vi "Insert Menu Items.vi"(6 "after item":string, 7 "menu tag":string, 8 "error in (no error)":errorcluster, 9 "item tags":string[](array[string]), 10 "item names":string[](array[string]), 11 "Menu in":refnum<class "Menu.lvclass">) -> (0 "error out":errorcluster, 1 "item tags out":string[](array[string]), 3 "Menu out":refnum<class "Menu.lvclass">)   [LabVIEW 2021, in "Menu.lvlib" / "Menu.lvclass"]
uses:
  Menu.lvclass
  <vilib>/Utility/miscctls.llb/LVMapReplaceAction.ctl
  <vilib>/Utility/miscctls.llb/LVPoint32TypeDef.ctl
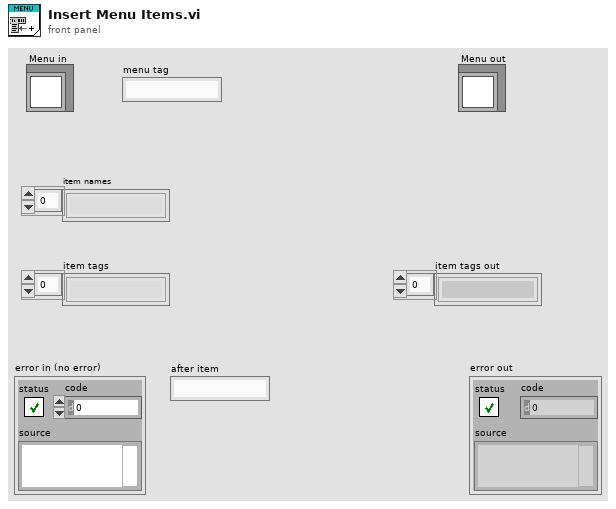
[diagram p1: front panel]
types:
  T1 = typedef "LVPoint32TypeDef.ctl" = cluster{"Horizontal":i32, "Vertical":i32}
  T2 = typedef "LVMapReplaceAction.ctl" = enum32{"Modify Entry only if found", "Add or Modify Entry", "Delete Entry"}
  T3 = typedef "Menu.lvlib/Menu.lvclass/Data.ctl" = cluster{"MenuMap":map{string, T4}, "PictRef":refnum<vi>, "MenuSelectionEvent":refnum<user-event>, "TopMenuSpacing":i32, "MenuSpacing":i32, "CloseEvent":refnum<user-event>, "TR_ManageMenuRef":refnum<vi>, "MenuColors":T6, "RTMPath":path, "RTMVIReference":refnum<vi>, "RTMMenuReference":refnum<k9>, "CtlRef":refnum<vi>, "User-Specified Font":refnum<class "Font.lvclass">, "Desired Font":enum16{"User-specified Font", "Application Font", "System Font", "Dialog Font"}, "SubMenuIcon":T7, "SubMenuIconClosed":refnum<class "Picture2D.lvclass">, "SubMenuIconOpened":refnum<class "Picture2D.lvclass">}
  T4 = typedef "Menu.lvlib/Menu.lvclass/MenuItems.ctl" = cluster{"Item Name":string, "Short Cut":T5, "Checked":bool, "Enable":bool, "After item":string, "Item Tags":string[], "Item Names":string[], "Picture":refnum<class "Image.lvclass">, "Hilite Picture":refnum<class "Image.lvclass">, "Displayed":bool}
  T5 = typedef "LVMenuShortCut.ctl" = cluster{"Include Shift Key?":bool, "Include Ctrl Key?":bool, "Shortcut Key":string}
  T6 = typedef "Menu.lvlib/Menu.lvclass/MenuColors.ctl" = cluster{"Text":refnum<class "Color.lvclass">, "HiliteText":refnum<class "Color.lvclass">, "Background":refnum<class "Color.lvclass">, "BorderColor":refnum<class "Color.lvclass">, "Hilite":refnum<class "Color.lvclass">}
  T7 = typedef "Menu.lvlib/Menu.lvclass/SubMenuIcon.ctl" = enum16{"LabVIEW", "Windows", "Custom"}
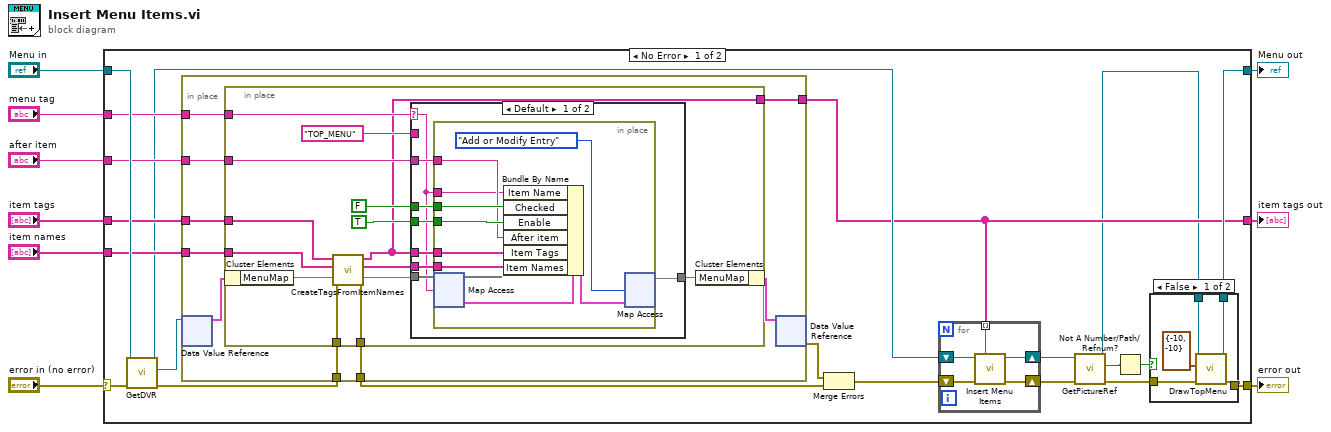
[diagram p0: block diagram]
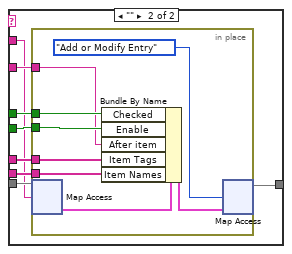
[diagram p3: hidden frame]
diagram:
  n1 = case shown="No Error" "error in (no error)" {
    selector: "error in (no error)" -> [w28 w100]
    tunnel: [w20 w100] -> w8
    tunnel: [w19 w99] -> w6
    tunnel: "Menu in" -> [w30 w99]
    tunnel: "menu tag" -> [w26 _]
    tunnel: "after item" -> [w25 _]
    tunnel: "item tags" -> [w24 w98]
    tunnel: "item names" -> [w23 _]
    tunnel: [w16 w98] -> w1
    frame No Error {
      n2 = call "GetDVR.vi"("error in (no error)"=w28, "Menu in"=w30) -> ("error out"=w22:errorcluster, "DVR"=w29:refnum<data-value>, "Menu out"=w17:refnum<class "Menu.lvclass">)  [unwired: 7 in]
      n3 = in-place {
        in-place-border: w26 -> [w49]
        in-place-border: w25 -> [w48]
        in-place-border: w24 -> [w47]
        in-place-border: w23 -> [w46]
        in-place-border: [w45] -> w16
        in-place-border: w22 -> [w44]
        in-place-border: [w43] -> w21
        n4 = in-place-dvr #1(w29) -> (w51:T3)  [unwired: 1 out]
        n5 = in-place {
          in-place-border: w49 -> [w63]
          in-place-border: w48 -> [w55]
          in-place-border: w47 -> [w62]
          in-place-border: w46 -> [w61]
          in-place-border: [w52] -> w45
          in-place-border: w44 -> [w59]
          in-place-border: [w58] -> w43
          n6 = in-place-cluster #2(w51) -> ("MenuMap"=w64:map{string, T4})
          n7 = call "CreateTagsFromItemNames.vi"("error in"=w59, "item names"=w61, "item tags"=w62) -> ("error out"=w58:errorcluster, "item names"=w54:string[], "item tags"=w52:string[])  [unwired: 6 in]
          n8 = case shown="Default" w63 {
            selector: w63 -> [w65 _]
            tunnel: w64 -> [w72 w89]
            tunnel: [w71 w88] -> w60
            tunnel: FALSE ("Checked") -> [w70 w87]
            tunnel: TRUE ("Enable") -> [w69 w86]
            tunnel: w55 -> [w68 w85]
            tunnel: w52 -> [w67 w84]
            tunnel: w54 -> [w66 w83]
            tunnel: "TOP_MENU" ("key") -> [_ w82]
            frame Default {
              n9 = in-place {
                in-place-border: w70 -> [w81]
                in-place-border: w69 -> [w80]
                in-place-border: w68 -> [w79]
                in-place-border: w67 -> [w78]
                in-place-border: w66 -> [w77]
                in-place-border: w65 -> [w73]
                n10 = in-place-map #3(w72, w65) -> (w76:T4)  [unwired: 1 in, 1 out]
                n11 = Bundle By Name(cluster=w76, "Item Name"=w73, "Checked"=w81, "Enable"=w80, "After item"=w79, "Item Tags"=w78, "Item Names"=w77) -> (w75:T4)
                n12 = in-place-map #3(w75, LVMapReplaceAction."Add or Modify Entry" ("action")) -> (w71:map{string, T4})  [unwired: 2 out]
              }
            }
            frame "" {
              n13 = in-place {
                in-place-border: w87 -> [w97]
                in-place-border: w86 -> [w96]
                in-place-border: w85 -> [w95]
                in-place-border: w84 -> [w94]
                in-place-border: w83 -> [w93]
                n14 = in-place-map #4(w89, w82) -> (w92:T4)  [unwired: 1 in, 1 out]
                n15 = Bundle By Name(cluster=w92, "Checked"=w97, "Enable"=w96, "After item"=w95, "Item Tags"=w94, "Item Names"=w93) -> (w91:T4)
                n16 = in-place-map #4(w91, LVMapReplaceAction."Add or Modify Entry" ("action")) -> (w88:map{string, T4})  [unwired: 2 out]
              }
            }
          }
          n17 = in-place-cluster #2("MenuMap"=w60) -> (w50:T3)
        }
        n18 = in-place-dvr #1(w50) -> (w27:errorcluster)  [unwired: 1 out]
      }
      n19 = Merge Errors(w27, w21) -> (w18:errorcluster)
      n20 = for {
        shift-right: [w39] -> w15
        shift-left: w18 -> [w42]
        shift-right: [w40] -> w13
        shift-left: w17 -> [w41]
        tunnel: w16 -> [w38] mode=indexing
        n21 = call "Insert Menu Items.vi"("menu tag"=w38, "error in (no error)"=w42, "Menu in"=w41) -> ("error out"=w39:errorcluster, "Menu out"=w40:refnum<class "Menu.lvclass">)  [unwired: 6 in, 1 out]
      }
      n22 = call "GetPictureRef.vi"("error in (no error)"=w15, "Menu in"=w13) -> ("error out"=w14:errorcluster, "PictRef"=w11:refnum<vi>, "Menu out"=w12:refnum<class "Menu.lvclass">)  [unwired: 7 in]
      n23 = Not A Number/Path/Refnum?(number/path/refnum=w11) -> (NaN/Path/Refnum?=w10:bool)
      n24 = case shown="False" w10 {
        tunnel: [w35 w37] -> w20
        tunnel: [w34 w36] -> w19
        tunnel: w12 -> [w32 w36]
        tunnel: w14 -> [w31 w37]
        frame False {
          n25 = call "DrawTopMenu.vi"("error in (no error)"=w31, "Coords"=T1 {"Horizontal"=-10, "Vertical"=-10}, "Menu in"=w32) -> ("error out"=w35:errorcluster, "Menu out"=w34:refnum<class "Menu.lvclass">)  [unwired: 4 in, 3 out]
        }
        frame True {
        }
      }
    }
    frame Error {
    }
  }
  "error out" <- w8
  "Menu out" <- w6
  "item tags out" <- w1
